vi "SIM921 Value.vi"(7 "Wait (ms)":u32=30, 8 "Error In":errorcluster, 9 "Query":string, 10 "Slot":T1(ring), 11 "VISA resource name":refnum<visa-resource-name>) -> (0 "Error Out":errorcluster, 1 "String Response":string, 2 "Resistance":dbl[](array[numeric]), 3 "VISA resource name":refnum<visa-resource-name>)   [LabVIEW 2021]
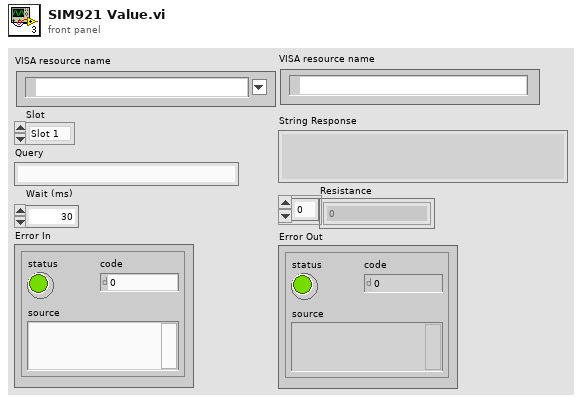
[diagram p1: front panel]
types:
  T1 = enum32{"Slot 1", "Slot 2", "Slot 3", "Slot 4", "Slot 5", "Slot 6", "Slot 7", "Slot 8"}
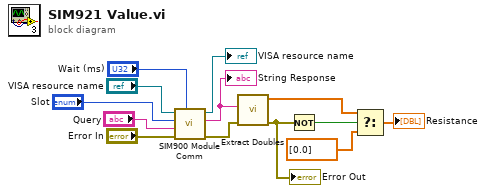
[diagram p0: block diagram]
diagram:
  n1 = call "SIM900 Module Comm.vi"("Wait (ms)"="Wait (ms)", "Error In"="Error In", "Query"="Query", "Slot"="Slot", "VISA Resource Name"="VISA resource name") -> ("Error Out"=w2:errorcluster, "Response"=w9:string, "dup VISA Session"=→"VISA resource name":refnum<visa-resource-name>)  [unwired: 4 in]
  "String Response" <- w9
  n2 = call "Extract Doubles.vi"("error in"=w2, "String"=w9) -> ("error out"=w1:errorcluster, "Data"=w11:dbl[])  [unwired: 4 in]
  "Error Out" <- w1
  n3 = Not(x=w1) -> (.not. x?=w10:bool)
  n4 = Select(t=w11, s=w10, f=dbl[] [0.0]) -> (s? t:f=→"Resistance":dbl[])
